vi "PPMSDR - Sweep control.vi"(0 "Scan control":cluster{"Priority":u16, "Scan name":u16}[](array[cluster])=[{"Priority"=1, "Scan name"=0}, {"Priority"=2, "Scan name"=0}, {"Priority"=0, "Scan name"=5}, {"Priority"=3, "Scan name"=0}] {"Scan name" items=["OFF", "Vsg1", "Vsg2", "Vsgw", "Vbg", "Field", "Temp", "MW_freq", "MW_amplitude"]; "Priority" items=["Priority 0", "Priority 1", "Priority 2", "Priority 3", "Priority 4", "Priority 5"]}, 1 "Scan parameters":T2(array[cluster])=[{"DAQ Channel"=2, "Label"="\nappliedVsg=", "Scaled low"=-0.1, "Scaled high"=0.6, "Start"=-0.05, "End"=0.25, "Step"=0.002, "Scale?"=FALSE}, {"DAQ Channel"=1, "Label"="\nappliedT=", "Scaled low"=-0.175, "Scaled high"=0.775, "Start"=0.07, "End"=0.4, "Step"=0.01, "Scale?"=FALSE}, {"DAQ Channel"=3, "Label"="\nappliedVsg=", "Scaled low"=-0.11, "Scaled high"=0.31, "Start"=-90000.0, "End"=90000.0, "Step"=1000.0, "Scale?"=FALSE}, {"DAQ Channel"=3, "Label"="\nappliedField=", "Scaled low"=-0.060000000000000005, "Scaled high"=0.14, "Start"=90000.0, "End"=-90000.0, "Step"=500.0, "Scale?"=FALSE}] {"Step" format="%#_6p"; "End" format="%#_6p"; "Start" format="%#_6p"; "Scaled high" format="%#_6p"; "Scaled low" format="%#_6p"}, 2 "Channels: AO 2":T1={"AO amp (V)"=[0.00075, 0.0, 0.0, 0.0], "AO DC (V)"=[0.00036, 0.0, 0.0, 0.0], "AO f (Hz)"=[0.4, 0.0, 0.0, 0.0], "AO phi (deg)"=[0.0, 0.0, 0.0, 0.0], "function"=[enum."Triangle Wave", enum."Sine Wave", enum."Sine Wave", enum."Sine Wave"]} {"AO DC (V)" format="%#_6p"; "AO amp (V)" format="%#_6p"}, 3 "Comments":string="B=-9T\nVsg sweep from -50mV to 250mV, 2mV step\nVbg =-1.1V\nTC=0.3s\n\nI+/-: 2/5 25uVac + 360uVdc 13 Hz\nV+/-: 3/4\nV2+/-: 1/26", 4 "Experiment folder name":string="3A - sweep Vsg @ -9T, IV") -> ()   [LabVIEW 2013]
panel:
  in  "set sg to inital value?":bool
  in  "Additional action (indexing priority)":u16[](array[ring])=[5, 5, 5, 5] items=["Clear DAQ Tasks", "Check Temperature", "Check Field Value", "Wait", "Temp Below X", "Do Nothing"]
  in  "Enum":enum16{"IV", "lockin", "IV/lockin continuous B"}(ring)=enum."lockin"
  in  "Number of IV curves":i32=1
  # "Instructions: \n1, you can put multiple scan names in one priority.\n2 OFF has to put in last priority"
  # "if you use the lockin\nprogram remember to\nset BG/SG parameters in\n'lockin_Vsg_multichannel.vi'"
  # "0"
  # "1"
  # "2"
  # "3"
  # "4"
  # "5"
  # "6"
  # "7"
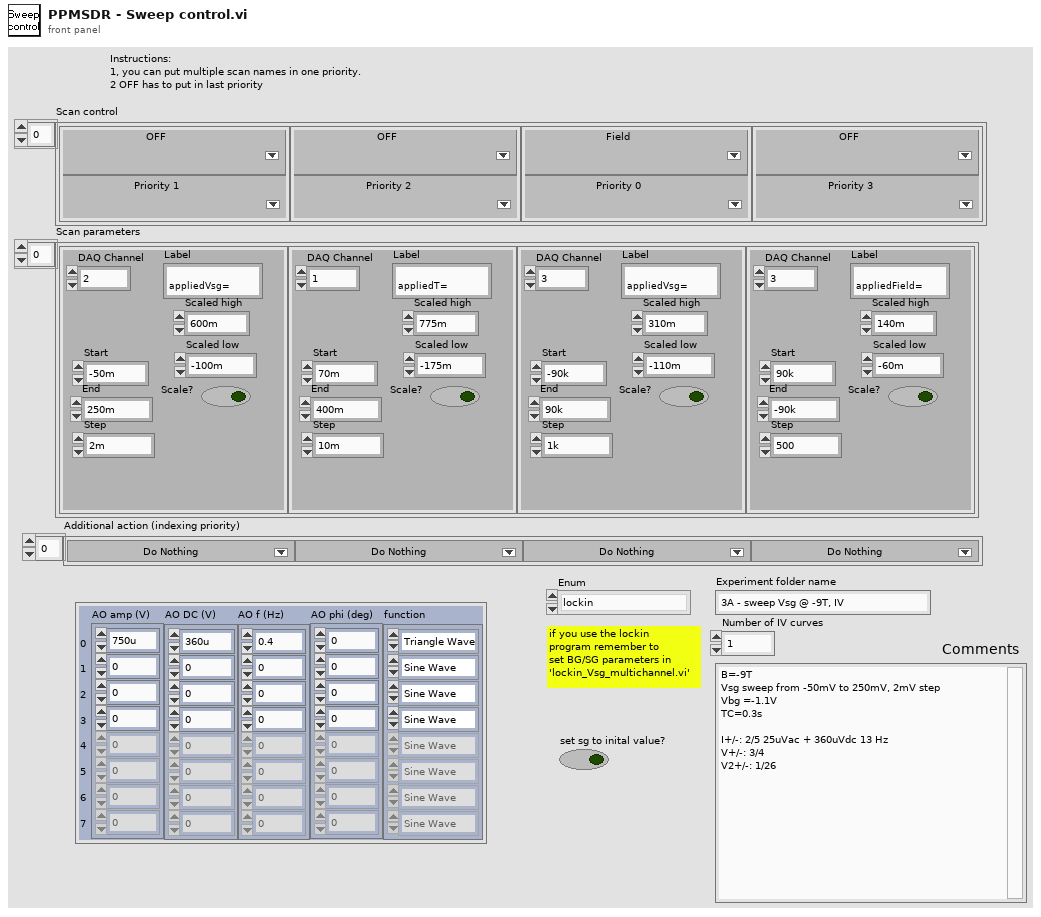
[diagram p1: front panel]
types:
  T1 = cluster{"AO amp (V)":dbl[], "AO DC (V)":dbl[], "AO f (Hz)":dbl[], "AO phi (deg)":dbl[], "function":enum16{"Sine Wave", "Triangle Wave", "Square Wave", "Sawtooth Wave"}[]}
  T2 = cluster{"DAQ Channel":i32, "Label":string, "Scaled low":dbl, "Scaled high":dbl, "Start":dbl, "End":dbl, "Step":dbl, "Scale?":bool}[]
  T3 = cluster{cluster{"DAQ Channel":i32, "Label":string, "Scaled low":dbl, "Scaled high":dbl, "Start":dbl, "End":dbl, "Step":dbl, "Scale?":bool}[]}[]
  T4 = cluster{cluster{"Priority":u16, "Scan name":u16}[]}[]
  T5 = cluster{cluster{"DAQ Channel":i32, "Label":string, "Scaled low":dbl, "Scaled high":dbl, "Start":dbl, "End":dbl, "Step":dbl, "Scale?":bool}[]}
  T6 = cluster{cluster{"Priority":u16, "Scan name":u16}[]}
  T7 = cluster{"DAQ Channel":i32, "Label":string, "Scaled low":dbl, "Scaled high":dbl, "Start":dbl, "End":dbl, "Step":dbl, "Scale?":bool}
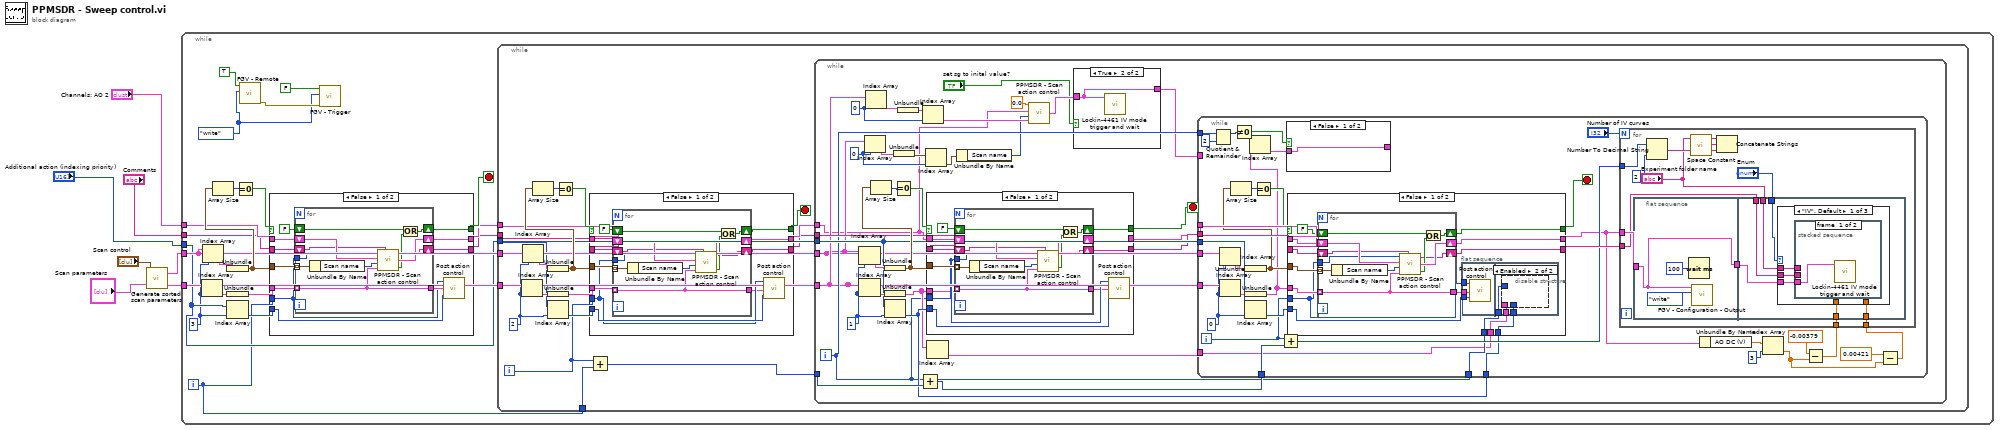
[diagram p0: block diagram]
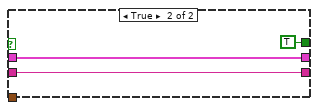
[diagram p2: hidden frame]
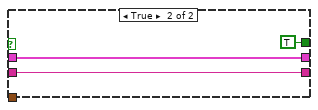
[diagram p3: hidden frame]
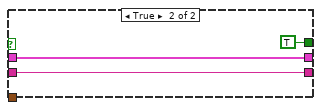
[diagram p5: hidden frame]
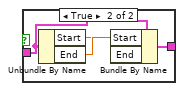
[diagram p6: hidden frame]
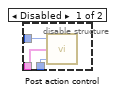
[diagram p7: hidden frame]
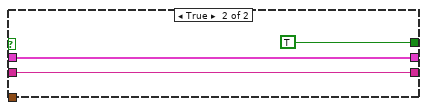
[diagram p8: hidden frame]
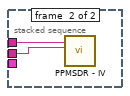
[diagram p9: hidden frame]
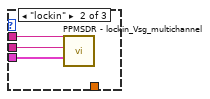
[diagram p10: hidden frame]
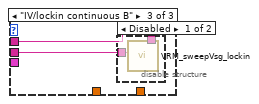
[diagram p11: hidden frame]
diagram:
  n1 = call <userlib>:"Generate sorted scan parameters.vi"("Scan parameters"="Scan parameters", "Scan control"="Scan control") -> ("Sorted scan parameters"=w3:T3, "Sorted scan control"=w4:T4)
  n2 = while {
    tunnel: "Comments" -> [w16]
    tunnel: "Channels: AO 2" -> [w17]
    tunnel: w3 -> [w23]
    tunnel: w4 -> [w22]
    tunnel: "Additional action (indexing priority)" -> [w18]
    i -> [w12]
    stop <- w20 stop-if-true
    w8 = enum16{"write", "read"}."write" ("Function")
    w13 = 3
    n3 = Index Array(array=w23, index=w13) -> (element=w24:T5)
    n4 = Index Array(array=w22, index=w13) -> (element=w21:T6)
    n5 = Unbundle(w21) -> (w26:cluster{"Priority":u16, "Scan name":u16}[])
    n6 = Array Size(array=w26) -> (size(s)=w27:i32)
    n7 = Unbundle(w24) -> (w25:T2)
    n8 = Index Array(array=w18, index=w13) -> (element=w19:u16)
    n9 = Equal To 0?(x=w27) -> (x = 0?=w28:bool)
    n10 = call <userlib>:"FGV - Remote.vi"("Function"=w8, "Remote Mode"=TRUE) -> ("error out"=w9:errorcluster)  [unwired: 4 in, 1 out]
    n11 = case shown="False" w28 {
      tunnel: w25 -> [w39 _]
      tunnel: [w38 w52] -> w15
      tunnel: [w37 w51] -> w14
      tunnel: [w31 TRUE ("Stop?")] -> w20
      tunnel: w26 -> [w36 _]
      tunnel: w12 -> [w33 _]
      tunnel: w19 -> [w34 _]
      tunnel: w17 -> [w30 w52]
      tunnel: w16 -> [w29 w51]
      frame False {
        n12 = for {
          tunnel: w36 -> [w50] mode=indexing
          tunnel: w39 -> [w47] mode=indexing
          tunnel: w33 -> [w44]
          shift-right: [w42] -> w38
          shift-left: w30 -> [w45]
          shift-right: [w40] -> w37
          shift-left: w29 -> [w43]
          tunnel: [w47] -> w35
          shift-right: [w48] -> w31
          shift-left: FALSE -> [w49]
          n13 = Unbundle By Name(w50) -> ("Scan name"=w46:u16)
          n14 = call <userlib>:"PPMSDR - Scan action control.vi"("Index"=w44, "Channels: AO"=w45, "Scan control"=w46, "Scan Parameters"=w47, "Comments"=w43) -> ("Comments out"=w40:string, "Channels: AO 2"=w42:T1, "Stop?"=w41:bool)
          n15 = Or(x=w49, y=w41) -> (x .or. y?=w48:bool)
        }
        n16 = call <userlib>:"Post action control.vi"("Action"=w34, "Scan Parameters"=w35, "Index"=w33) -> ()  [unwired: 1 out]
      }
      frame True {
      }
    }
    n17 = call <userlib>:"FGV - Trigger.vi"("error in"=w9, "Function"=w8, "Trigger"=FALSE) -> ()  [unwired: 3 in, 2 out]
    n18 = while {
      tunnel: w23 -> [w65]
      tunnel: w22 -> [w64]
      tunnel: w18 -> [w63]
      tunnel: w14 -> [w62]
      tunnel: w15 -> [w61]
      tunnel: w12 -> [w55]
      i -> [w56]
      stop <- w60 stop-if-true
      w57 = 2
      n19 = Index Array(array=w65, index=w57) -> (element=w71:T5)
      n20 = Index Array(array=w64, index=w57) -> (element=w72:T6)
      n21 = Unbundle(w72) -> (w69:cluster{"Priority":u16, "Scan name":u16}[])
      n22 = Array Size(array=w69) -> (size(s)=w67:i32)
      n23 = Unbundle(w71) -> (w70:T2)
      n24 = Index Array(array=w63, index=w57) -> (element=w68:u16)
      n25 = Equal To 0?(x=w67) -> (x = 0?=w66:bool)
      n26 = case shown="False" w66 {
        tunnel: w70 -> [w78 _]
        tunnel: w61 -> [w81 w97]
        tunnel: w62 -> [w80 w96]
        tunnel: [w75 w97] -> w59
        tunnel: [w74 w96] -> w58
        tunnel: [w76 TRUE ("Stop?")] -> w60
        tunnel: w69 -> [w79 _]
        tunnel: w56 -> [w77 _]
        tunnel: w68 -> [w83 _]
        frame False {
          n27 = for {
            tunnel: w79 -> [w94] mode=indexing
            tunnel: w78 -> [w91] mode=indexing
            tunnel: w77 -> [w88]
            shift-right: [w86] -> w75
            shift-left: w81 -> [w89]
            shift-right: [w84] -> w74
            shift-left: w80 -> [w87]
            tunnel: [w91] -> w73
            shift-right: [w92] -> w76
            shift-left: FALSE -> [w93]
            n28 = Unbundle By Name(w94) -> ("Scan name"=w90:u16)
            n29 = call <userlib>:"PPMSDR - Scan action control.vi"("Index"=w88, "Channels: AO"=w89, "Scan control"=w90, "Scan Parameters"=w91, "Comments"=w87) -> ("Comments out"=w84:string, "Channels: AO 2"=w86:T1, "Stop?"=w85:bool)
            n30 = Or(x=w93, y=w85) -> (x .or. y?=w92:bool)
          }
          n31 = call <userlib>:"Post action control.vi"("Action"=w83, "Scan Parameters"=w73, "Index"=w77) -> ()  [unwired: 1 out]
        }
        frame True {
        }
      }
      n32 = Add(x=w56, y=w55) -> (x+y=w54:i32)
      n33 = while {
        tunnel: w59 -> [w102]
        tunnel: w58 -> [w125]
        tunnel: w64 -> [w111]
        tunnel: w65 -> [w113]
        tunnel: w63 -> [w124]
        tunnel: w54 -> [w119]
        i -> [w114]
        stop <- w121 stop-if-true
        w105 = 0 ("index")
        w108 = 0 ("index")
        w120 = 1
        n34 = Index Array(array=w111, index=w120) -> (element=w126:T6)
        n35 = Index Array(array=w113, index=w120) -> (element=w127:T5)
        n36 = Index Array(array=w111, index=w105) -> (element=w110:T6)
        n37 = Index Array(array=w113, index=w108) -> (element=w112:T5)
        n38 = Unbundle(w126) -> (w128:cluster{"Priority":u16, "Scan name":u16}[])
        n39 = Array Size(array=w128) -> (size(s)=w129:i32)
        n40 = Unbundle(w127) -> (w116:T2)
        n41 = Index Array(array=w124, index=w120) -> (element=w117:u16)
        n42 = Equal To 0?(x=w129) -> (x = 0?=w130:bool)
        n43 = Unbundle(w110) -> (w106:cluster{"Priority":u16, "Scan name":u16}[])
        n44 = Unbundle(w112) -> (w109:T2)
        n45 = Add(x=w114, y=w119) -> (x+y=w118:i32)
        n46 = Index Array(array=w109, index=w108) -> (element=w107:T7)
        n47 = Index Array(array=w106, index=w105) -> (element=w104:cluster{"Priority":u16, "Scan name":u16})
        n48 = case shown="False" w130 {
          tunnel: w116 -> [w137 _]
          tunnel: w102 -> [w141 w157]
          tunnel: w125 -> [w140 w156]
          tunnel: [w135 w157] -> w122
          tunnel: [w134 w156] -> w123
          tunnel: [w136 TRUE ("Stop?")] -> w121
          tunnel: w128 -> [w139 _]
          tunnel: w114 -> [w138 _]
          tunnel: w117 -> [w143 _]
          frame False {
            n49 = for {
              tunnel: w139 -> [w154] mode=indexing
              tunnel: w137 -> [w151] mode=indexing
              tunnel: w138 -> [w148]
              shift-right: [w146] -> w135
              shift-left: w141 -> [w149]
              shift-right: [w144] -> w134
              shift-left: w140 -> [w147]
              tunnel: [w151] -> w133
              shift-right: [w152] -> w136
              shift-left: FALSE -> [w153]
              n50 = Unbundle By Name(w154) -> ("Scan name"=w150:u16)
              n51 = call <userlib>:"PPMSDR - Scan action control.vi"("Index"=w148, "Channels: AO"=w149, "Scan control"=w150, "Scan Parameters"=w151, "Comments"=w147) -> ("Comments out"=w144:string, "Channels: AO 2"=w146:T1, "Stop?"=w145:bool)
              n52 = Or(x=w153, y=w145) -> (x .or. y?=w152:bool)
            }
            n53 = call <userlib>:"Post action control.vi"("Action"=w143, "Scan Parameters"=w133, "Index"=w138) -> ()  [unwired: 1 out]
          }
          frame True {
          }
        }
        n54 = Index Array(array=w116) -> (element=w115:T7)  [unwired: 1 in]
        n55 = Unbundle By Name(w104) -> ("Scan name"=w103:u16)
        n56 = call <userlib>:"PPMSDR - Scan action control.vi"("Index"=0.0, "Channels: AO"=w102, "Scan control"=w103, "Scan Parameters"=w107) -> ("Channels: AO 2"=w101:T1)  [unwired: 1 in, 2 out]
        n57 = case shown="True" "set sg to inital value?" {
          tunnel: w101 -> [w131 w132]
          tunnel: [w131 w132] -> w98
          frame False {
          }
          frame True {
            n58 = call <userlib>:"Lockin-4461 IV mode trigger and wait.vi"("Channels: AO"=w132) -> ()  [unwired: 10 in, 1 out]
          }
        }
        n59 = while {
          tunnel: w111 -> [w191]
          tunnel: w113 -> [w190]
          tunnel: w122 -> [w187]
          tunnel: w123 -> [w186]
          tunnel: w124 -> [w183]
          tunnel: w118 -> [w178]
          tunnel: w117 -> [w175]
          tunnel: w114 -> [w176]
          tunnel: w115 -> [w174]
          tunnel: w114 -> [w171]
          tunnel: w98 -> [_]
          i -> [w167]
          stop <- w184 stop-if-true
          w180 = 0
          n60 = Quotient & Remainder(x=w171, y=2) -> (x-y*floor(x/y)=w169:i32)  [unwired: 1 out]
          n61 = Index Array(array=w191, index=w180) -> (element=w189:T6)
          n62 = Index Array(array=w190, index=w180) -> (element=w188:T5)
          n63 = Not Equal To 0?(x=w169) -> (x != 0?=w168:bool)
          n64 = Unbundle(w189) -> (w173:cluster{"Priority":u16, "Scan name":u16}[])
          n65 = Array Size(array=w173) -> (size(s)=w182:i32)
          n66 = Unbundle(w188) -> (w166:T2)
          n67 = Index Array(array=w183, index=w180) -> (element=w179:u16)
          n68 = Index Array(array=w166) -> (element=w172:T7)  [unwired: 1 in]
          n69 = Equal To 0?(x=w182) -> (x = 0?=w181:bool)
          n70 = Add(x=w167, y=w178) -> (x+y=w177:i32)
          n71 = case shown="False" w168 {
            tunnel: w172 -> [w193 w197]
            tunnel: [w193 w194] -> _
            frame False {
            }
            frame True {
              n72 = Unbundle By Name(w197) -> ("Start"=w195:dbl, "End"=w196:dbl)
              n73 = Bundle By Name(cluster=w197, "Start"=w196, "End"=w195) -> (w194:T7)
            }
          }
          n74 = case shown="False" w181 {
            tunnel: w166 -> [w206 _]
            tunnel: w187 -> [w209 w234]
            tunnel: w186 -> [w208 w233]
            tunnel: [w203 w234] -> w165
            tunnel: [w202 w233] -> w185
            tunnel: [w204 TRUE ("Stop?")] -> w184
            tunnel: w173 -> [w207 _]
            tunnel: w167 -> [w205 _]
            tunnel: w179 -> [w211 _]
            tunnel: w176 -> [w198 _]
            tunnel: w175 -> [w200 _]
            tunnel: w174 -> [w199 _]
            frame False {
              n75 = for {
                tunnel: w207 -> [w231] mode=indexing
                tunnel: w206 -> [w228] mode=indexing
                tunnel: w205 -> [w225]
                shift-right: [w223] -> w203
                shift-left: w209 -> [w226]
                shift-right: [w221] -> w202
                shift-left: w208 -> [w224]
                tunnel: [w228] -> w201
                shift-right: [w229] -> w204
                shift-left: FALSE -> [w230]
                n76 = Unbundle By Name(w231) -> ("Scan name"=w227:u16)
                n77 = call <userlib>:"PPMSDR - Scan action control.vi"("Index"=w225, "Channels: AO"=w226, "Scan control"=w227, "Scan Parameters"=w228, "Comments"=w224) -> ("Comments out"=w221:string, "Channels: AO 2"=w223:T1, "Stop?"=w222:bool)
                n78 = Or(x=w230, y=w222) -> (x .or. y?=w229:bool)
              }
              n79 = flat-sequence {
                tunnel: w211 -> [w214]
                tunnel: w205 -> [w213]
                tunnel: w201 -> [w212]
                tunnel: w200 -> [w217]
                tunnel: w199 -> [w216]
                tunnel: w198 -> [w215]
                frame #0 {
                  n80 = call <userlib>:"Post action control.vi"("Action"=w214, "Scan Parameters"=w212, "Index"=w213) -> ()  [unwired: 1 out]
                }
                frame #1 {
                  n81 = disable-structure shown="Enabled" {
                    disable-tunnel: w217 -> [w220 _]
                    disable-tunnel: w216 -> [w219 _]
                    disable-tunnel: w215 -> [w218 _]
                    frame Disabled {
                      n82 = call <userlib>:"Post action control.vi"("Action"=w220, "Scan Parameters"=w219, "Index"=w218) -> ()  [unwired: 1 out]
                    }
                    frame Enabled {
                    }
                  }
                }
              }
            }
            frame True {
            }
          }
          n83 = Unbundle By Name(w165) -> ("AO DC (V)"=w162:dbl[])
          n84 = Index Array(array=w162, index=3) -> (element=w160:dbl)
          n85 = Subtract(x=-0.00379 ("Vmin (start)"), y=w160) -> (x-y=w163:dbl)
          n86 = Subtract(x=0.00421 ("Vmax (end)"), y=w160) -> (x-y=w158:dbl)
          n87 = for {
            N: "Number of IV curves" -> [_]
            tunnel: w165 -> [w245]
            tunnel: w185 -> [w239]
            tunnel: w177 -> [w243]
            tunnel: w163 -> [w236]
            tunnel: w158 -> [w235]
            n88 = flat-sequence {
              tunnel: w245 -> [w246]
              tunnel: [w246] -> w237
              tunnel: "Enum" -> [w250]
              tunnel: w239 -> [w254]
              tunnel: "Experiment folder name" -> [w249]
              tunnel: w236 -> [w253]
              tunnel: w235 -> [w252]
              tunnel: w237 -> [w251]
              frame #0 {
                n89 = Wait (ms)(milliseconds to wait=u32 100) -> ()  [unwired: 1 out]
                n90 = call <userlib>:"FGV - Configuration - Output.vi"("Function"=enum16{"write", "read"}."write", "Channels: AO"=w246) -> ()  [unwired: 4 in, 2 out]
              }
              frame #1 {
                n91 = case shown="\"IV\", Default" w250 {
                  tunnel: w254 -> [w256 w262 w264]
                  tunnel: w249 -> [w255 w263 w265]
                  tunnel: w251 -> [w257 w261 _]
                  tunnel: w253 -> [_ _ _]
                  tunnel: w252 -> [_ _ _]
                  frame "IV", Default {
                    n92 = stacked-sequence {
                      tunnel: w257 -> [w258 _]
                      tunnel: w256 -> [_ w260]
                      tunnel: w255 -> [_ w259]
                      frame #0 {
                        n93 = call <userlib>:"Lockin-4461 IV mode trigger and wait.vi"("Channels: AO"=w258) -> ()  [unwired: 10 in, 1 out]
                      }
                      frame #1 {
                        n94 = call "PPMSDR - IV.vi"("Notes"=w260, "Experiment folder name"=w259) -> ()  [unwired: 10 in]
                      }
                    }
                  }
                  frame "lockin" {
                    n95 = call "PPMSDR - lockin_Vsg_multichannel.vi"("Channels: AO"=w261, "Comments"=w262, "ITX folder"=w263) -> ()  [unwired: 9 in]
                  }
                  frame "IV/lockin continuous B" {
                    n96 = disable-structure shown="Disabled" {
                      disable-tunnel: w265 -> [w267 _]
                      disable-tunnel: w264 -> [w266 _]
                      frame Disabled {
                        n97 = call "VRM_sweepVsg_lockin.vi"("Comments"=w266, "ITX folder"=w267) -> ()  [unwired: 7 in, 1 out]
                      }
                      frame Enabled {
                      }
                    }
                  }
                }
              }
            }
            n98 = Number To Decimal String(number=w243, width (-)=i16 2) -> (decimal integer string=w242:string)
            n99 = call <vilib>:"Space Constant.vi"() -> ("String"=w241:string)
            n100 = Concatenate Strings("Experiment folder name", w241, w242) -> ()  [unwired: 1 out]
          }
        }
      }
    }
  }
